vi "remove list channel to configuration.vi"(8 "error in (no error)":errorcluster, 9 "element name":string, 10 "node ref":refnum<data-value>, 11 "engine ref":refnum<data-value>) -> (0 "error out":errorcluster)   [LabVIEW 2014, in "Shared Memory editor node.lvclass"]
uses:
  Shared Memory editor node.lvclass
  <vilib>/NI/DCAF/Tag Editor Core/Configuration Editor/Classes/Module editor node/module editor node.lvclass
  <vilib>/NI/DCAF/Tag Editor Core/Configuration Editor/Classes/Engine Parent/Engine Parent Editor Node.lvclass
  <vilib>/NI/Tag Bus/tag/tag descriptor.lvclass/tag descriptor.ctl
  <vilib>/NI/Configuration Framework/serializable configuration/NISE_CEF_serializable configuration.lvclass/NISE_CEF_serializable configuration.ctl
  <vilib>/Utility/LVClass/Get LV Class Name.vi
  <vilib>/NI/Configuration Framework/error generator/NISE_error generator.vi
  module/configuration/Shared Memory configuration.lvclass
  <vilib>/NI/Configuration Framework/serializable configuration/NISE_CEF_serializable configuration.lvclass
  <vilib>/NI/Tag Bus/tag/tag descriptor.lvclass
  <vilib>/NI/Module Execution Interface/Engine Configuration/engine configuration.lvclass
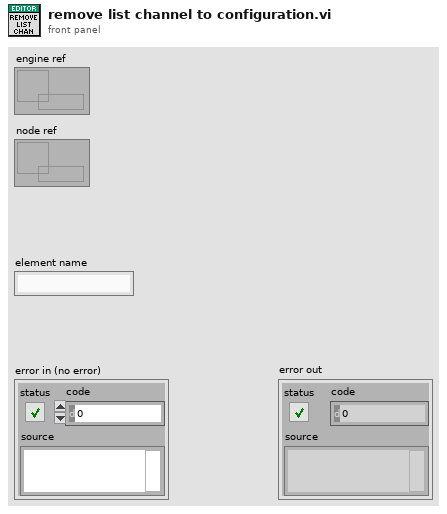
[diagram p1: front panel]
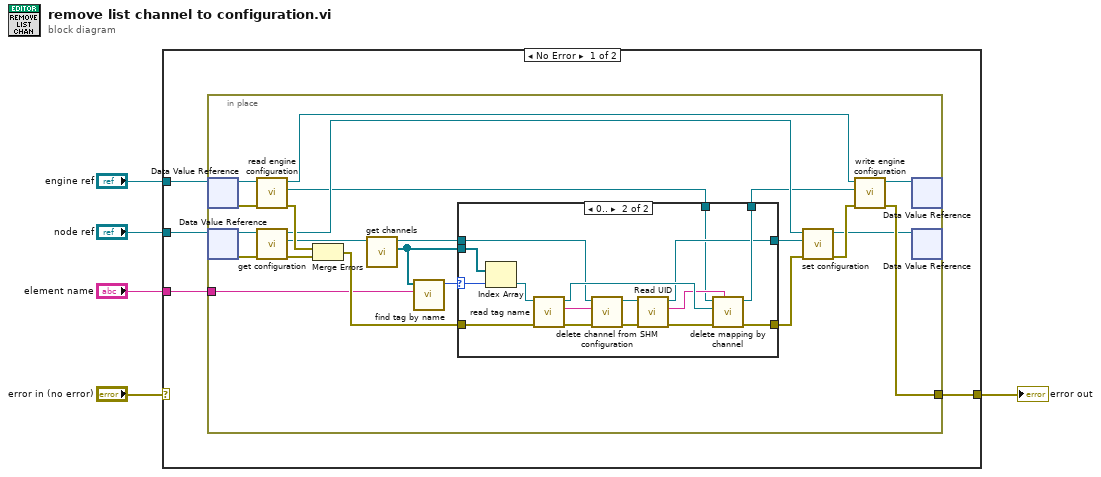
[diagram p0: block diagram]
diagram:
  n1 = case shown="No Error" "error in (no error)" {
    selector: "error in (no error)" -> [_ w51]
    tunnel: "node ref" -> [w9 _]
    tunnel: "engine ref" -> [w8 _]
    tunnel: "element name" -> [w7 _]
    tunnel: [w6 w51] -> w1
    frame No Error {
      n2 = in-place {
        in-place-border: w7 -> [w14]
        in-place-border: [w22] -> w6
        # "Replace the C header file directory destination in the module configuration."
        n3 = in-place-dvr #1(w8) -> (w31:refnum<class "Engine Parent Editor Node.lvclass">, w28:errorcluster)
        n4 = in-place-dvr #2(w9) -> (w29:refnum<class "module editor node.lvclass">, w26:errorcluster)
        n5 = call <vilib>:"read engine configuration.vi"("error in"=w28, "Engine Parent Editor Node in"=w31) -> ("error out"=w27:errorcluster, "engine configuration"=w20:refnum<class "engine configuration.lvclass">, "Engine Parent Editor Node out"=w24:refnum<class "Engine Parent Editor Node.lvclass">)  [unwired: 7 in]
        n6 = call "get configuration.vi"("error in (no error)"=w26, "shared memory editor node in"=w29) -> ("error out"=w25:errorcluster, "shm configuration out"=w18:refnum<class "Shared Memory configuration.lvclass">, "shared memory editor node out"=w21:refnum<class "module editor node.lvclass">)  [unwired: 7 in]
        n7 = Merge Errors(w27, w25) -> (w15:errorcluster)
        n8 = call-dynamic "get channels.vi"("Shared Memory configuration in"=w18) -> ("channels"=w11:refnum<class "TBM channel.lvclass">[], "Shared Memory configuration out"=w17:refnum<class "Shared Memory configuration.lvclass">)  [unwired: 9 in]
        n9 = call <vilib>:"find tag by name.vi"("name"=w14, "tags in"=w11) -> ("index"=w16:i32)  [unwired: 9 in]
        n10 = case shown="0.." w16 {
          selector: w16 -> [_ w50]
          tunnel: w17 -> [w34 w36]
          tunnel: [w34 w44] -> w13
          tunnel: [w33 w48] -> w12
          tunnel: w15 -> [w33 w41]
          tunnel: [w32 w49] -> w19
          tunnel: w11 -> [_ w35]
          tunnel: w20 -> [w32 w42]
          frame ..-1 {
          }
          frame 0.. {
            n11 = Index Array(array=w35, index=w50) -> (element=w47:refnum<class "TBM channel.lvclass">)
            n12 = call <vilib>:"read tag name.vi"("error in"=w41, "system tag in"=w47) -> ("error out"=w40:errorcluster, "name"=w38:string, "system tag out"=w46:refnum<class "TBM channel.lvclass">)  [unwired: 7 in]
            n13 = call "delete channel from SHM configuration.vi"("error in"=w40, "channel to delete"=w38, "SHM configuration in"=w36) -> ("error out"=w39:errorcluster, "SHM configuration out"=w37:refnum<class "Shared Memory configuration.lvclass">)  [unwired: 7 in]
            n14 = call <vilib>:"Read UID.vi"("error in"=w39, "configuration in"=w37) -> ("error out"=w45:errorcluster, "instance id"=w43:string, "configuration out"=w44:refnum<class "Shared Memory configuration.lvclass">)  [unwired: 7 in]
            n15 = call <vilib>:"delete mapping by channel.vi"("owner ID"=w43, "error in"=w45, "channel"=w46, "engine configuration in"=w42) -> ("error out"=w48:errorcluster, "engine configuration out"=w49:refnum<class "engine configuration.lvclass">)  [unwired: 6 in]
          }
        }
        n16 = call "set configuration.vi"("error in (no error)"=w12, "shm configuration in"=w13, "shared memory editor node in"=w21) -> ("error out"=w23:errorcluster, "shared memory editor node out"=w10:refnum<class "module editor node.lvclass">)  [unwired: 7 in]
        n17 = call <vilib>:"write engine configuration.vi"("error in"=w23, "engine configuration"=w19, "Engine Parent Editor Node in"=w24) -> ("error out"=w22:errorcluster, "Engine Parent Editor Node out"=w30:refnum<class "Engine Parent Editor Node.lvclass">)  [unwired: 7 in]
        n18 = in-place-dvr #1(w30) -> ()  [unwired: 2 out]
        n19 = in-place-dvr #2(w10) -> ()  [unwired: 2 out]
      }
    }
    frame Error {
    }
  }
  "error out" <- w1
